vi "FL_Make_Track_overlay_DAQmx.vi"(4 "Rainbow track is speed (F)":bool, 5 "Speed array":dbl[](array[numeric]), 6 "Full track array":T2(array[cluster]), 7 "Colors array input":u32[](array[colorbox]), 8 "Image In":T1) -> (3 "Image Out":T1)   [LabVIEW 2018, in "Tracker.lvlib"]
uses:
  Tracker.lvlib
  <vilib>/vision/Image Controls.llb/IMAQ Image.ctl
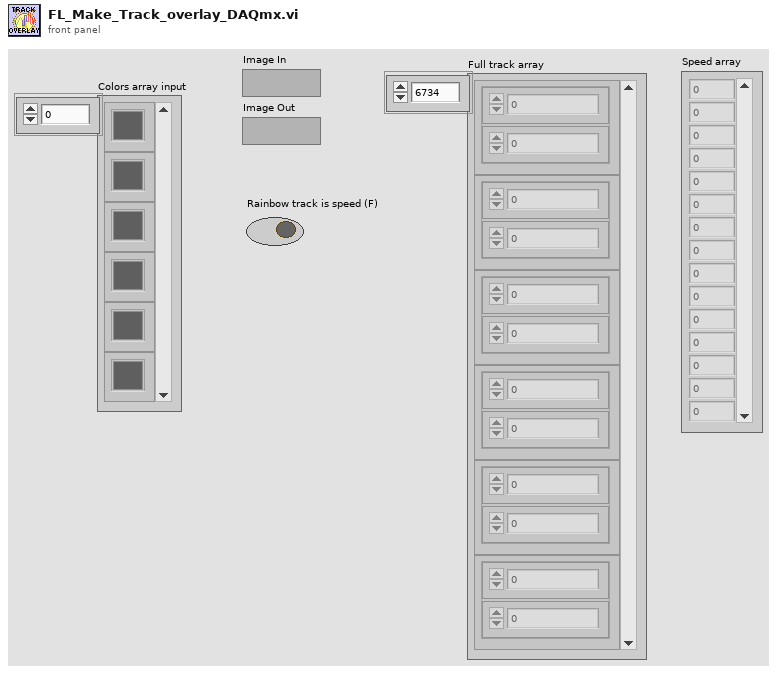
[diagram p1: front panel]
types:
  T1 = typedef "IMAQ Image.ctl" = refnum<image>
  T2 = cluster{"Numeric Control":dbl, "Numeric Control":dbl}[]
  T3 = cluster{"Numeric Control":dbl, "Numeric Control":dbl}
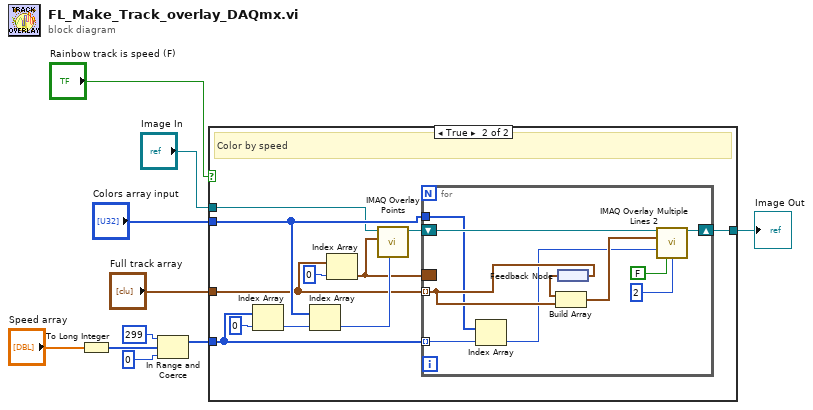
[diagram p0: block diagram]
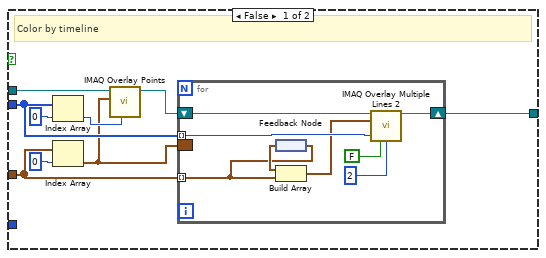
[diagram p2: hidden frame]
diagram:
  n1 = To Long Integer(number="Speed array") -> (32bit integer=w4:i32[])
  n2 = In Range and Coerce(upper limit=299, x=w4, lower limit=0) -> (coerced(x)=w1:i32[])  [unwired: 1 out]
  n3 = case shown="True" "Rainbow track is speed (F)" {
    tunnel: "Colors array input" -> [w19 w38]
    tunnel: "Full track array" -> [w16 w36]
    tunnel: "Image In" -> [w14 w34]
    tunnel: [w11 w31] -> w7
    tunnel: w1 -> [_ w28]
    frame False {
      # "Color by timeline"
      n4 = Index Array(array=w19, index=0) -> (element=w17:u32)
      n5 = Index Array(array=w16, index=0) -> (element=w12:T3)
      n6 = call "IMAQ Overlay Points"("Color"=w17, "Point"=w12, "Image"=w14) -> ("Image Out"=w13:T1)  [unwired: 7 in, 1 out]
      n7 = for {
        shift-right: [w27] -> w11
        shift-left: w13 -> [w21]
        tunnel: w16 -> [w23] mode=indexing
        tunnel: w19 -> [w26] mode=indexing
        border: w12 -> [_]
        n8 = feedback-in #1(w23) -> ()
        n9 = feedback #1() -> (w24:T3)
        n10 = Build Array(w24, w23) -> (w22:T2)
        n11 = call "IMAQ Overlay Multiple Lines 2"("Image"=w21, "Line End Points"=w22, "Color"=w26, "Maintain Width?"=FALSE, "Width"=u32 2) -> ("Image Out"=w27:T1)  [unwired: 9 in, 1 out]
      }
    }
    frame True {
      # "Color by speed"
      n12 = Index Array(array=w28, index=0) -> (element=w29:i32)
      n13 = Index Array(array=w38, index=w29) -> (element=w37:u32)
      n14 = Index Array(array=w36, index=0) -> (element=w32:T3)
      n15 = call "IMAQ Overlay Points"("Color"=w37, "Point"=w32, "Image"=w34) -> ("Image Out"=w33:T1)  [unwired: 7 in, 1 out]
      n16 = for {
        shift-right: [w48] -> w31
        shift-left: w33 -> [w43]
        tunnel: w36 -> [w45] mode=indexing
        tunnel: w38 -> [w41]
        border: w32 -> [_]
        tunnel: w28 -> [w40] mode=indexing
        n17 = Index Array(array=w41, index=w40) -> (element=w39:u32)
        n18 = feedback-in #2(w45) -> ()
        n19 = feedback #2() -> (w46:T3)
        n20 = Build Array(w46, w45) -> (w44:T2)
        n21 = call "IMAQ Overlay Multiple Lines 2"("Image"=w43, "Line End Points"=w44, "Color"=w39, "Maintain Width?"=FALSE, "Width"=u32 2) -> ("Image Out"=w48:T1)  [unwired: 9 in, 1 out]
      }
    }
  }
  "Image Out" <- w7
